vi "TestExec.Config, Get Station SW Module Info.vi"(7 "Error if EXE does not exist":bool, 8 "Error if File Doesn't Exist":bool, 9 "Create File if Doesn't Exist":bool, 11 "Path":path=path "C:/MTE/Test Executive/Config") -> (0 "error out":errorcluster, 1 "Station IP Port":i32, 2 "Station Name":string, 3 "Sta Exe Path":path)   [LabVIEW 2019]
uses:
  <vilib>/Utility/config.llb/Read Key (String).vi
  <vilib>/Utility/config.llb/Read Key (I32).vi
  <vilib>/Utility/config.llb/Read Key (Path).vi
  <vilib>/KATE/Files/File Utils.lvlib
  <vilib>/Utility/config.llb/NI_LVConfig.lvlib
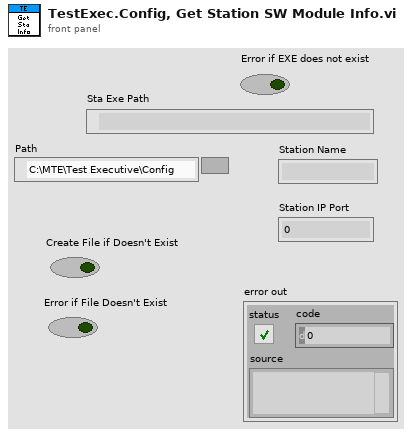
[diagram p1: front panel]
types:
  T1 = cluster{"Sta App":path, "Station Config":path, "ListenPort":u32, "Sta Name":string, "Station Folder":path}
  T2 = typedef "NI_LVConfig.lvlib/Config Data RefNum.ctl" = refnum<k1>
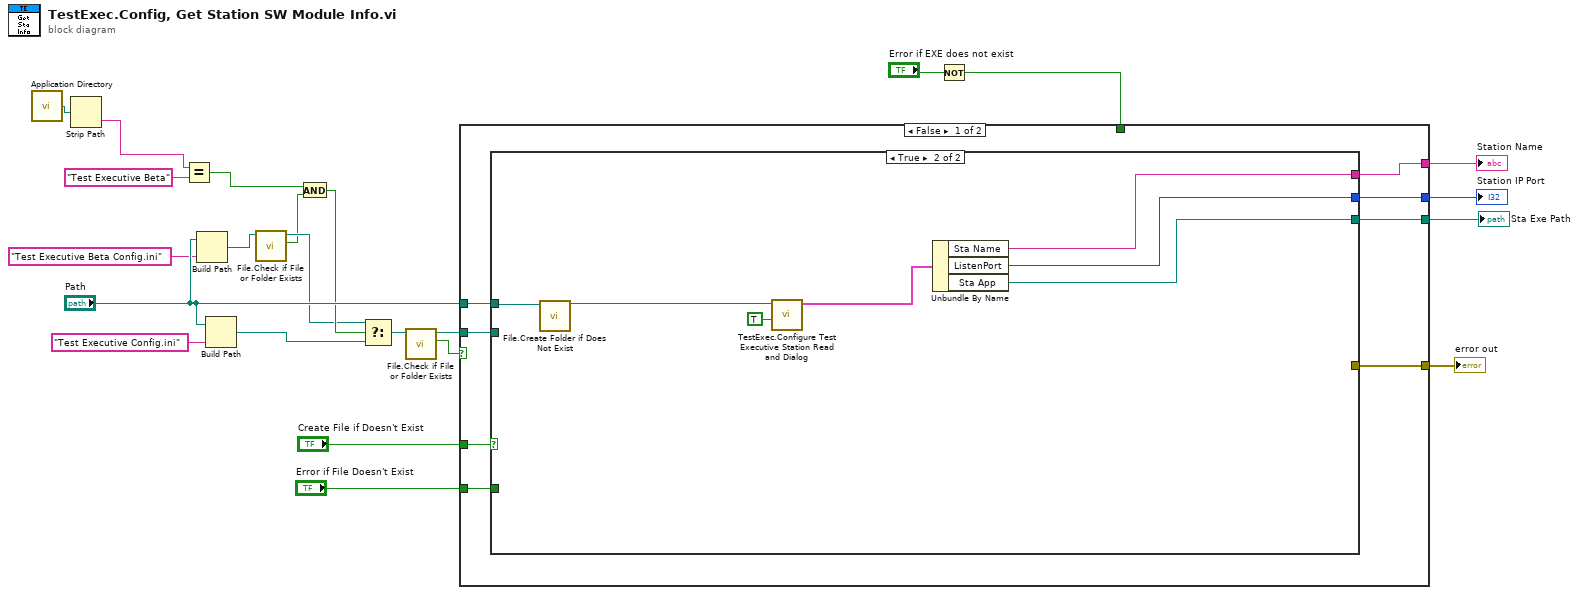
[diagram p0: block diagram]
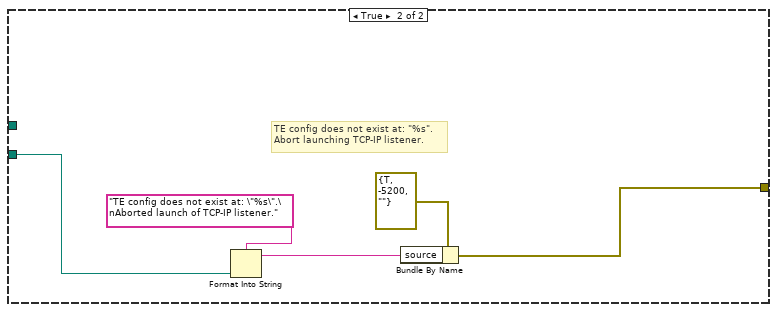
[diagram p3: hidden frame]
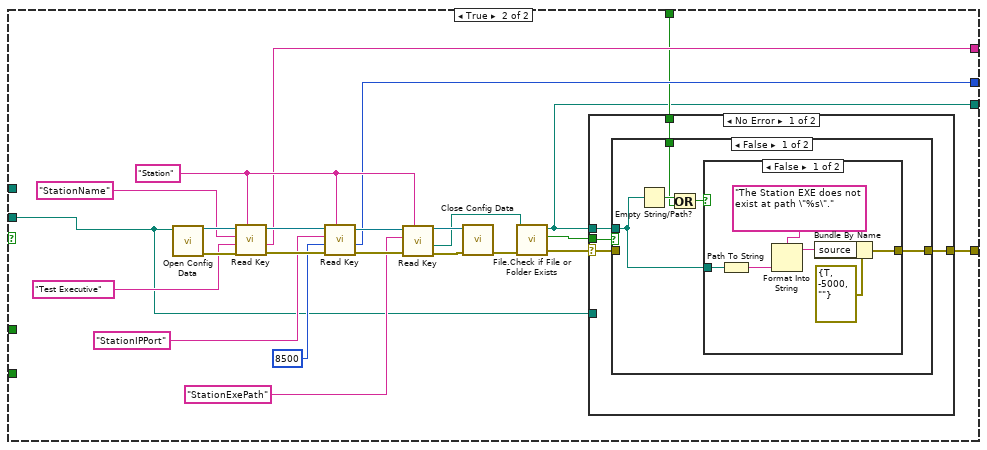
[diagram p4: hidden frame]
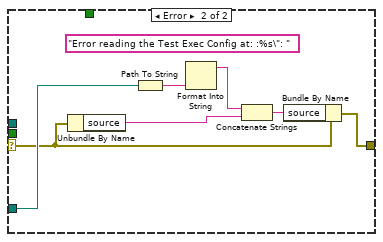
[diagram p7: hidden frame]
diagram:
  n1 = call <vilib>:"Application Directory.vi"() -> ("Application Directory"=w2:path)
  n2 = Strip Path(path=w2) -> (name=w1:string)  [unwired: 1 out]
  n3 = Equal?(x=w1, y="Test Executive Beta") -> (x = y?=w11:bool)
  n4 = Build Path(base path="Path", name or relative path="Test Executive Beta Config.ini") -> (appended path=w9:path)
  n5 = Build Path(base path="Path", name or relative path="Test Executive Config.ini") -> (appended path=w4:path)
  n6 = call <vilib>:"File.Check if File or Folder Exists.vi"("Path"=w9) -> ("Exists"=w6:bool, "Dup Path"=w7:path)  [unwired: 6 in, 3 out]
  n7 = And(x=w11, y=w6) -> (x .and. y?=w8:bool)
  n8 = Select(t=w7, s=w8, f=w4) -> (s? t:f=w5:path)
  n9 = call <vilib>:"File.Check if File or Folder Exists.vi"("Path"=w5) -> ("Exists"=w20:bool, "Dup Path"=w21:path)  [unwired: 6 in, 3 out]
  n10 = Not(x="Error if EXE does not exist") -> (.not. x?=w14:bool)
  n11 = case shown="False" w20 {
    tunnel: [w31 w68] -> w23
    tunnel: w21 -> [w26 w52]
    tunnel: "Create File if Doesn't Exist" -> [w30 _]
    tunnel: [w28 w51] -> w18
    tunnel: [w29 w50] -> w17
    tunnel: "Error if File Doesn't Exist" -> [w27 _]
    tunnel: "Path" -> [w25 _]
    tunnel: w14 -> [_ w49]
    tunnel: [w24 w48] -> w13
    frame False {
      n12 = case shown="True" w30 {
        tunnel: [w33 _] -> w31
        tunnel: [_ w42] -> w29
        tunnel: [_ w43] -> w28
        tunnel: w27 -> [w35 _]
        tunnel: w26 -> [w34 _]
        tunnel: w25 -> [w32 w47]
        tunnel: [_ w41] -> w24
        frame False {
          n13 = case shown="False" w35 {
            tunnel: w34 -> [_ w39]
            tunnel: [_ w36] -> w33
            tunnel: w32 -> [_ _]
            frame False {
            }
            frame True {
              # "TE config does not exist at: \"%s\".\nAbort launching TCP-IP listener."
              n14 = Format Into String(format string="TE config does not exist at: \"%s\".\nAborted launch of TCP-IP listener." ("source"), w39) -> (resulting string=w37:string)  [unwired: 2 in, 1 out]
              n15 = Bundle By Name(cluster=errorcluster {"status"=TRUE, "code"=-5200, "source"=""} ("error constant"), "source"=w37) -> (w36:errorcluster)
            }
          }
        }
        frame True {
          n16 = call <vilib>:"File.Create Folder if Does Not Exist.vi"("Path"=w47) -> ("Dup Path"=w46:path)  [unwired: 8 in, 2 out]
          n17 = call "TestExec.Configure Test Executive Station Read and Dialog.vi"("Dialog"=TRUE, "TE Config Folder"=w46) -> ("Config Out"=w44:T1)  [unwired: 8 in, 1 out]
          n18 = Unbundle By Name(w44) -> ("Sta Name"=w43:string, "ListenPort"=w42:u32, "Sta App"=w41:path)
        }
      }
    }
    frame True {
      w58 = "Station" ("section")
      n19 = call <vilib>:"Open Config Data.vi"("configuration file path"=w52) -> ("error out"=w66:errorcluster, "refnum"=w67:T2)  [unwired: 8 in, 1 out]
      n20 = call-poly <vilib>:"Read Key.vi"("section"=w58, "error in (no error)"=w66, "default value"="Test Executive" ("section"), "key"="StationName" ("section"), "refnum"=w67) -> ("error out"=w65:errorcluster, "value"=w51:string, "refnum out"=w64:T2)  [unwired: 3 in, 1 out]
      n21 = call-poly <vilib>:"Read Key.vi"("section"=w58, "error in (no error)"=w65, "default value"=8500, "key"="StationIPPort", "refnum"=w64) -> ("error out"=w61:errorcluster, "value"=w50:i32, "refnum out"=w62:T2)  [unwired: 3 in, 1 out]
      n22 = call-poly <vilib>:"Read Key.vi"("section"=w58, "error in (no error)"=w61, "key"="StationExePath", "refnum"=w62) -> ("error out"=w60:errorcluster, "value"=w54:path, "refnum out"=w59:T2)  [unwired: 4 in, 1 out]
      n23 = call <vilib>:"Close Config Data.vi"("error in (no error)"=w60, "refnum"=w59) -> ("error out"=w71:errorcluster)  [unwired: 8 in, 1 out]
      n24 = call <vilib>:"File.Check if File or Folder Exists.vi"("error in"=w71, "Path"=w54) -> ("error out"=w70:errorcluster, "Exists"=w69:bool, "Dup Path"=w48:path)  [unwired: 5 in, 2 out]
      n25 = case shown="No Error" w70 {
        selector: w70 -> [w74 w90]
        tunnel: w69 -> [w76 _]
        tunnel: w48 -> [w75 _]
        tunnel: [w73 w89] -> w68
        tunnel: w52 -> [_ w94]
        tunnel: w49 -> [w72 _]
        frame No Error {
          n26 = case shown="False" w76 {
            tunnel: w75 -> [w80 _]
            tunnel: w74 -> [_ w88]
            tunnel: [w81 w88] -> w73
            tunnel: w72 -> [w77 _]
            frame False {
              n27 = Empty String/Path?(string/path=w80) -> (empty?=w79:bool)
              n28 = Or(x=w79, y=w77) -> (x .or. y?=w78:bool)
              n29 = case shown="False" w78 {
                tunnel: [w83 _] -> w81
                tunnel: w80 -> [w82 _]
                frame False {
                  n30 = Path To String(path=w82) -> (string=w87:string)
                  n31 = Format Into String(format string="The Station EXE does not exist at path \"%s\".", w87) -> (resulting string=w85:string)  [unwired: 2 in, 1 out]
                  n32 = Bundle By Name(cluster=errorcluster {"status"=TRUE, "code"=-5000, "source"=""} ("error constant"), "source"=w85) -> (w83:errorcluster)
                }
                frame True {
                }
              }
            }
            frame True {
            }
          }
        }
        frame Error {
          (unwired) "Error reading the Test Exec Config at: :%s\": "
          n33 = Unbundle By Name(w90) -> ("source"=w92:string)
          n34 = Path To String(path=w94) -> (string=w95:string)
          n35 = Format Into String(w95) -> (resulting string=w93:string)  [unwired: 3 in, 1 out]
          n36 = Concatenate Strings(w93, w92) -> (w91:string)
          n37 = Bundle By Name(cluster=w90, "source"=w91) -> (w89:errorcluster)
        }
      }
    }
  }
  "error out" <- w23
  "Station Name" <- w18
  "Station IP Port" <- w17
  "Sta Exe Path" <- w13
